vi "FXP Read base.vi"(8 "error in (no error)":errorcluster, 9 "data in":dbl, 10 "integersize":i32, 11 "shared variable refnum in":refnum<k21>) -> (0 "error out":errorcluster, 1 "data out":dbl, 3 "shared variable refnum out":refnum<k21>)   [LabVIEW 2015]
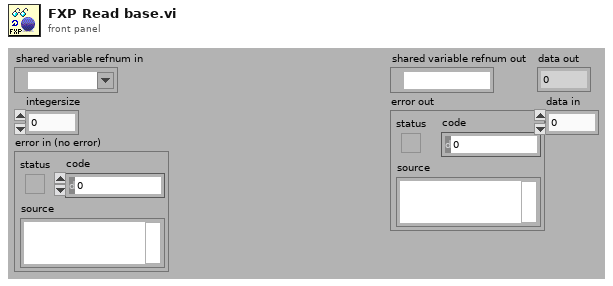
[diagram p1: front panel]
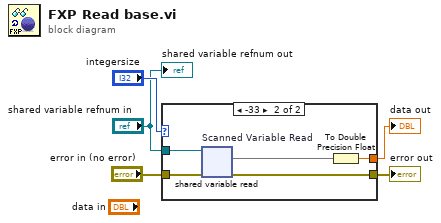
[diagram p0: block diagram]
diagram:
  n1 = case shown="-33" "integersize" {
    tunnel: "error in (no error)" -> [w6 w11]
    tunnel: [w6 w10] -> w3
    tunnel: "shared variable refnum in" -> [_ w9]
    tunnel: [_ w7] -> w1
    frame 2048, Default {
    }
    frame -33 {
      n2 = shared-variable-read "Scanned Variable Read"(w9, w11) -> (w10:errorcluster, w8)  [unwired: 1 in, 2 out]
      n3 = To Double Precision Float(number=w8) -> (double precision float=w7:dbl)
    }
  }
  "error out" <- w3
  "data out" <- w1
  "shared variable refnum out" <- "shared variable refnum in"
